vi "PlotScopeData.vi"() -> ()   [LabVIEW 2019]
uses:
  Motion/EnableSingle.vi
  Motion/MoveIncSingle.vi
panel:
  out "Waveform Chart":waveform(dbl)[](graph)
  in  "Number of points":i32=100 min=1 step=1
  in  "period":dbl=0.005 min=0.0001 max=1000.0
  in  "distance":dbl=5.0
  in  "speed":dbl=25.0
  in  "axisName":string="X"
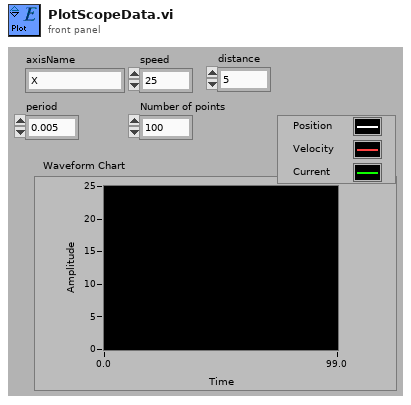
[diagram p1: front panel]
types:
  T1 = typedef "ControllerDataResults.ctl" = cluster{"AxisCount":i32, "DataPoints":i32, "ProgramCounter":i32[], "Axes":T2[]}
  T2 = typedef "AxisDataResults.ctl" = cluster{"Analog Input 0":dbl[], "Analog Input 1":dbl[], "Analog Output 0":dbl[], "Analog Output 1":dbl[], "Collection Rate":dbl, "Acceleration Command":dbl[], "Position Command":dbl[], "Velocity Command":dbl[], "Count":i32, "Current Command":sgl[], "Current Error":sgl[], "Current Feedback":sgl[], "Digital Input 0":i32[], "Digital Input 1":i32[], "Digital Input 2":i32[], "Digital Output 0":i32[], "Digital Output 1":i32[], "Digital Output 2":i32[], "Position Feedback Auxiliary":dbl[], "Position Feedback":dbl[], "Velocity Feedback":dbl[], "Optional Data 1":dbl[], "Optional Data 2":dbl[], "Position Error":dbl[], "Velocity Error":dbl[]}
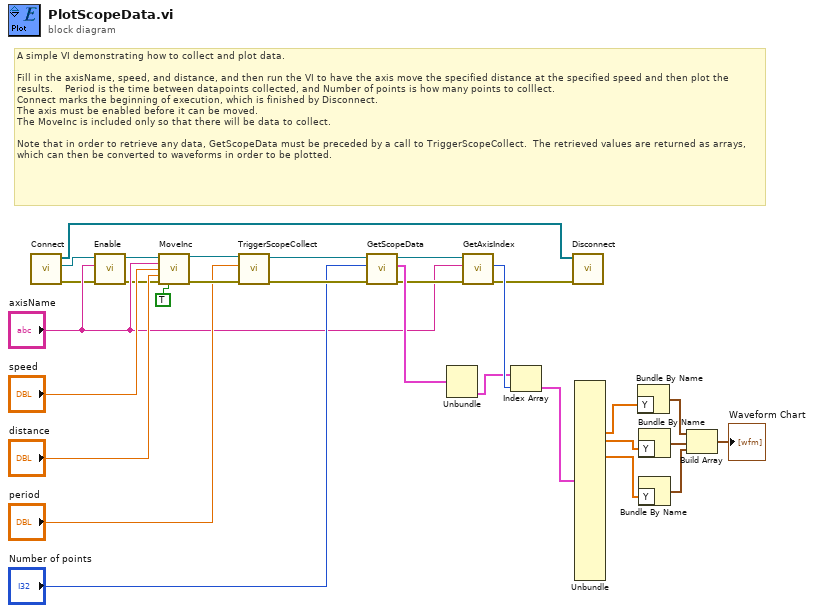
[diagram p0: block diagram]
diagram:
  # "A simple VI demonstrating how to collect and plot data.\n\nFill in the axisName, speed, and distance, and then run the VI to have the axis move the specified distance at the specified speed and then plot the results.    Period is the time between datapoints collected, and Number of points is how many points to colllect.\nConnect marks the beginning of execution, which is finished by Disconnect.\nThe axis must be enabled before it can be moved.\nThe MoveInc is included only so that there will be data to collect.\n\nNote that in order to retrieve any data, GetScopeData must be preceded by a call to TriggerScopeCollect.  The retrieved values are returned as arrays, which can then be converted to waveforms in order to be plotted."
  n1 = call "Connect.vi"() -> ("error out"=w5:errorcluster, "controller"=w7:refnum<k24>, "controllers"=w8:refnum<k24>[])  [unwired: 9 in]
  n2 = call-poly "Enable.vi"("error in (no error)"=w5, "axis name"="axisName", "controller in"=w7) -> ("error out"=w4:errorcluster, "controller out"=w3:refnum<k24>)  [unwired: 7 in]
  n3 = call-poly "MoveInc.vi"("controller in"=w3, "axis name"="axisName", "speed"="speed", "distance"="distance", "error in (no error)"=w4, "return immediately"=TRUE) -> ("controller out"=w27:refnum<k24>, "error out"=w26:errorcluster)  [unwired: 8 in]
  n4 = call "TriggerScopeCollect.vi"("error in (no error)"=w26, "period"="period", "controller in"=w27) -> ("error out"=w24:errorcluster, "controller out"=w25:refnum<k24>)  [unwired: 7 in]
  n5 = call "GetScopeData.vi"("error in (no error)"=w24, "number of points"="Number of points", "controller in"=w25) -> ("error out"=w19:errorcluster, "scope data"=w21:T1, "controller out"=w20:refnum<k24>)  [unwired: 6 in]
  n6 = Unbundle(w21) -> ("Axes"=w9:T2[])  [unwired: 3 out]
  n7 = call "GetAxisIndex.vi"("error in (no error)"=w19, "axis name"="axisName", "controller in"=w20) -> ("error out"=w1:errorcluster, "axis index"=w18:i32)  [unwired: 6 in, 1 out]
  n8 = Index Array(array=w9, index=w18) -> (element=w17:T2)
  n9 = call "Disconnect.vi"("error in (no error)"=w1, "controllers"=w8) -> ()  [unwired: 9 in, 1 out]
  n10 = Unbundle(w17) -> ("Position Command"=w12:dbl[], "Velocity Command"=w11:dbl[], "Current Command"=w10:sgl[])  [unwired: 22 out]
  n11 = Bundle By Name("Y"=w12) -> (w16:waveform(dbl))  [unwired: 1 in]
  n12 = Bundle By Name("Y"=w11) -> (w15:waveform(dbl))  [unwired: 1 in]
  n13 = Bundle By Name("Y"=w10) -> (w14:waveform(sgl))  [unwired: 1 in]
  n14 = Build Array(w16, w15, w14) -> (→"Waveform Chart":waveform(dbl)[])
